vi "JK.vi"() -> ()   [LabVIEW 2018]
panel:
  out "Z1":bool
  out "Z0":bool
  out "Q0":bool
  out "Q1":bool
  in  "stop":bool
  in  "Y":bool
  in  "X":bool
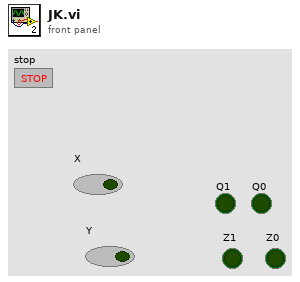
[diagram p1: front panel]
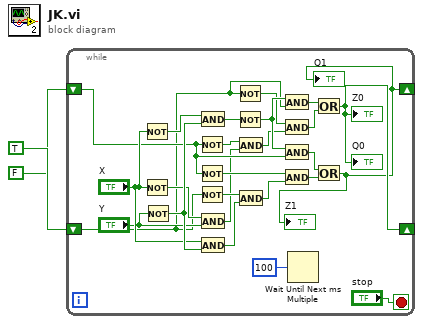
[diagram p0: block diagram]
diagram:
  n1 = while {
    shift-right: [w4] -> _
    shift-left: TRUE -> [w8]
    shift-right: [w3] -> _
    shift-left: FALSE -> [w13]
    stop <- "stop" stop-if-true
    n2 = Not(x="X") -> (.not. x?=w25:bool)
    n3 = Not(x="X") -> (.not. x?=w16:bool)
    n4 = Not(x="Y") -> (.not. x?=w24:bool)
    n5 = Not(x=w13) -> (.not. x?=w12:bool)
    n6 = Not(x=w13) -> (.not. x?=w22:bool)
    n7 = Not(x=w8) -> (.not. x?=w26:bool)
    n8 = And(x=w25, y=w24) -> (x .and. y?=w23:bool)
    n9 = And(x=w16, y="Y") -> (x .and. y?=w11:bool)
    n10 = And(x="X", y=w24) -> (x .and. y?=w27:bool)
    n11 = Not(x=w8) -> (.not. x?=w9:bool)
    n12 = Not(x=w23) -> (.not. x?=w10:bool)
    n13 = And(x=w12, y=w11) -> (x .and. y?=w7:bool)
    n14 = And(x=w26, y=w27) -> (x .and. y?=w21:bool)
    n15 = And(x=w10, y=w8) -> (x .and. y?=w6:bool)
    n16 = And(x=w9, y=w7) -> (x .and. y?=w5:bool)
    n17 = And(x=w10, y=w13) -> (x .and. y?=w20:bool)
    n18 = And(x=w22, y=w21) -> (x .and. y?=w19:bool)
    n19 = Wait Until Next ms Multiple(millisecond multiple=u32 100) -> ()  [unwired: 1 out]
    n20 = Or(x=w6, y=w5) -> (x .or. y?=w4:bool)
    "Q0" <- w4
    "Z0" <- w4
    n21 = Or(x=w20, y=w19) -> (x .or. y?=w3:bool)
    "Z1" <- w3
    "Q1" <- w3
  }
